vi "ReadDataUV-visSD_test.vi"(0 "Nombre de aq":i32=2, 1 "task out":refnum<k21> caption="tâche") -> (2 "Channel I":i32[][](array[numeric]), 3 "Channel II":i32[][](array[numeric]), 4 "DLL error code":u32=20066, 5 "temps d'acqu ms":u32=4148)   [LabVIEW 2015]
uses:
  dependecies/Error Code Enum typedef.ctl
  <vilib>/DAQmx/write.llb/DAQmx Write (Digital Bool 1Line 1Point).vi
panel:
  in  "Binning Horizontal":i32=1
  out "status":T1=enum."DRV_IDLE"
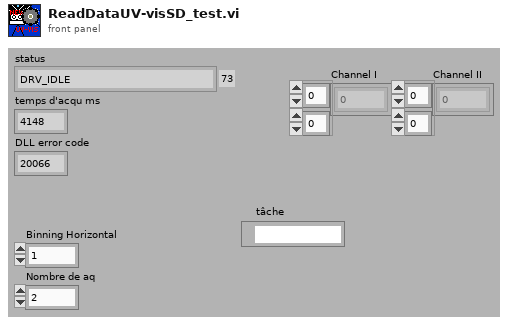
[diagram p1: front panel]
types:
  T1 = typedef "Error Code Enum typedef.ctl" = enum32{"N/A (0)", "DRV_ERROR_CODES", "DRV_SUCCESS", "DRV_VXDNOTINSTALLED", "DRV_ERROR_SCAN", "DRV_ERROR_CHECK_SUM", "DRV_ERROR_FILELOAD", "DRV_UNKNOWN_FUNC", "DRV_ERROR_VXD_INIT", "DRV_ERROR_ADDRESS", "DRV_ERROR_PAGELOCK", "DRV_ERROR_PAGEUNLOCK", "DRV_ERROR_BOARDTEST", "DRV_ERROR_ACK", "DRV_ERROR_UP_FIFO", "DRV_ERROR_PATTERN", "N/A (16)", "DRV_ACQUISITION_ERRORS", "DRV_ACQ_BUFFER", "DRV_ACQ_DOWNFIFO_FULL", "DRV_PROC_UNKONWN_INSTRUCTION", "DRV_ILLEGAL_OP_CODE", "DRV_KINETIC_TIME_NOT_MET", "DRV_ACCUM_TIME_NOT_MET", "DRV_NO_NEW_DATA", "N/A (25)", "DRV_SPOOLERROR", "N/A (27)", "N/A (28)", "N/A (29)", "N/A (30)", "N/A (31)", "N/A (32)", "DRV_TEMPERATURE_CODES", "DRV_TEMPERATURE_OFF", "DRV_TEMPERATURE_NOT_STABILIZED", "DRV_TEMPERATURE_STABILIZED", "DRV_TEMPERATURE_NOT_REACHED", "DRV_TEMPERATURE_OUT_RANGE", "DRV_TEMPERATURE_NOT_SUPPORTED", "DRV_TEMPERATURE_DRIFT", "N/A (41)", "N/A (42)", "N/A (43)", "N/A (44)", "N/A (45)", "N/A (46)", "N/A (47)", "N/A (48)", "DRV_GENERAL_ERRORS", "DRV_INVALID_AUX", "DRV_COF_NOTLOADED", "DRV_FPGAPROG", "DRV_FLEXERROR", "DRV_GPIBERROR", "N/A (55)", "N/A (56)", "N/A (57)", "N/A (58)", "N/A (59)", "N/A (60)", "N/A (61)", "N/A (62)", "N/A (63)", "DRV_DATATYPE", "DRV_DRIVER_ERRORS", "DRV_P1INVALID", "DRV_P2INVALID", "DRV_P3INVALID", "DRV_P4INVALID", "DRV_INIERROR", "DRV_COFERROR", "DRV_ACQUIRING", "DRV_IDLE", "DRV_TEMPCYCLE", "DRV_NOT_INITIALIZED", "DRV_P5INVALID", "DRV_P6INVALID", "DRV_INVALID_MODE", "DRV_INVALID_FILTER", "DRV_I2CERRORS", "DRV_I2CDEVNOTFOUND", "DRV_I2CTIMEOUT", "DRV_P7INVALID", "N/A (84)", "N/A (85)", "N/A (86)", "N/A (87)", "N/A (88)", "N/A (89)", "DRV_IOCERROR", "DRV_VRMVERSIONERROR"}
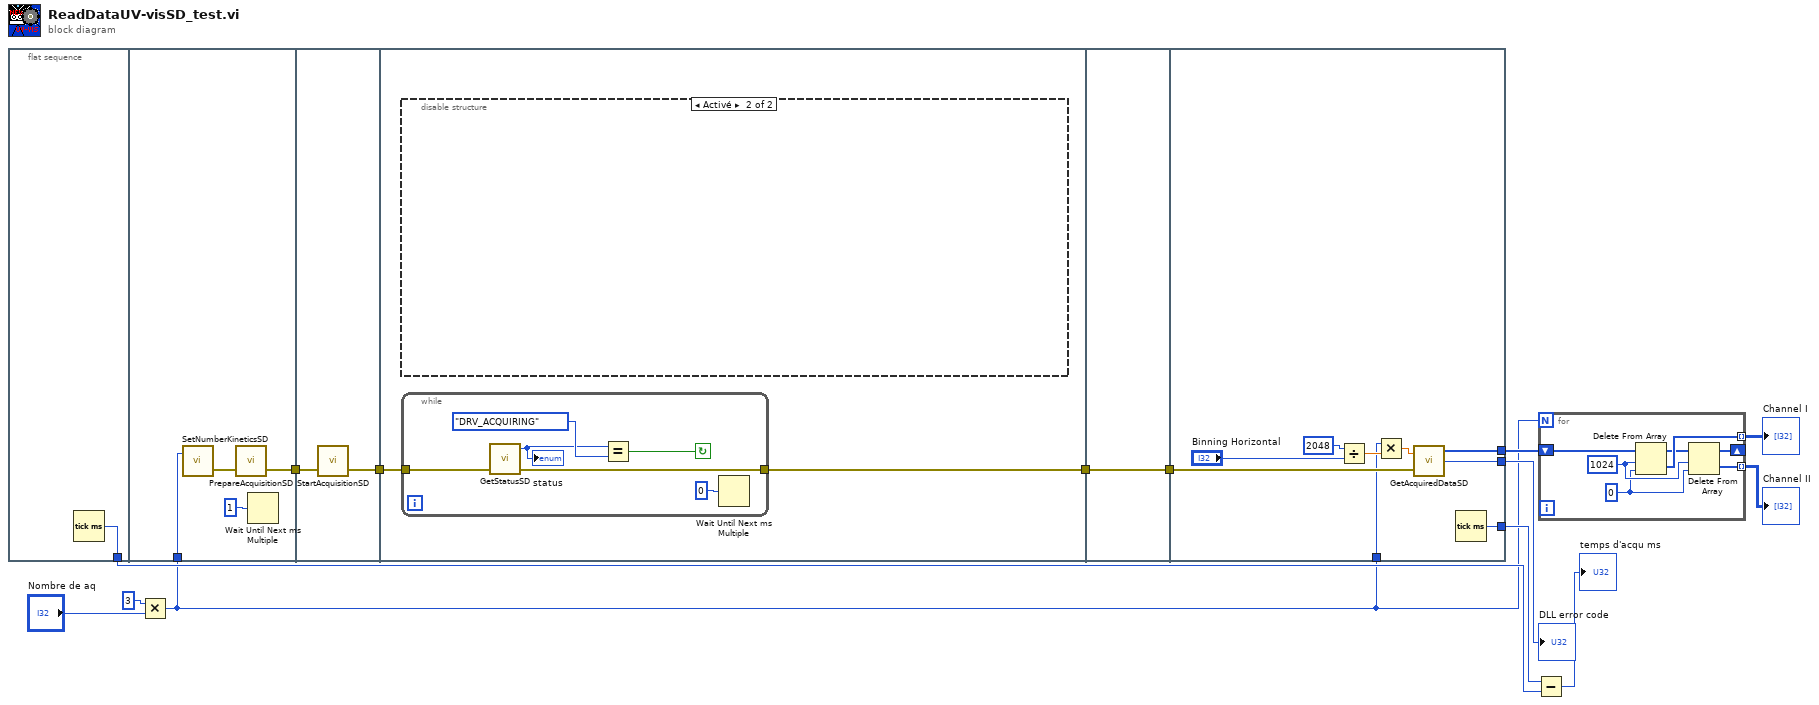
[diagram p0: block diagram]
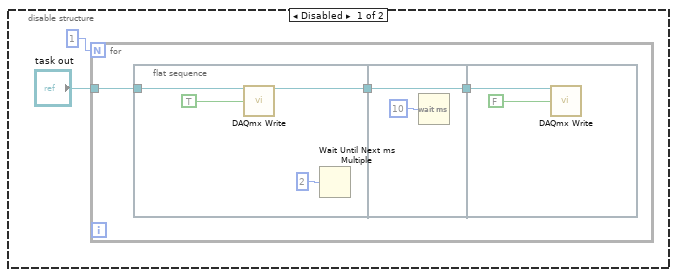
[diagram p2: hidden frame]
diagram:
  n1 = flat-sequence {
    tunnel: [w15] -> w10
    tunnel: [w17] -> w12
    tunnel: w2 -> [w16]
    tunnel: w12 -> [w21]
    tunnel: [w20] -> w11
    tunnel: w11 -> [w23]
    tunnel: [w22] -> w4
    tunnel: w4 -> [w43]
    tunnel: [w43] -> w3
    tunnel: [w51] -> w8
    tunnel: [w50] -> w14
    tunnel: w3 -> [w47]
    tunnel: [w46] -> w9
    tunnel: w2 -> [w45]
    frame #0 {
      n2 = Tick Count (ms)() -> (millisecond timer value=w15:u32)
    }
    frame #1 {
      n3 = call "SetNumberKineticsSD.vi"("number"=w16) -> ("error out"=w19:errorcluster)  [unwired: 1 in, 1 out]
      n4 = call "PrepareAcquisitionSD.vi"("error in (no error)"=w19) -> ("error out"=w17:errorcluster)  [unwired: 1 in, 1 out]
      n5 = Wait Until Next ms Multiple(millisecond multiple=u32 1 ("n millisecondes")) -> ()  [unwired: 1 out]
    }
    frame #2 {
      n6 = call "StartAcquisitionSD.vi"("error in (no error)"=w21) -> ("error out"=w20:errorcluster)  [unwired: 1 in, 1 out]
    }
    frame #3 {
      n7 = disable-structure shown="Activé" {
        frame Disabled {
          n8 = for {
            N: 1 -> [_]
            tunnel: "task out" -> [w28]
            n9 = flat-sequence {
              tunnel: w28 -> [w32]
              tunnel: [w30] -> w26
              tunnel: [w33] -> w27
              tunnel: w26 -> [w33]
              tunnel: w27 -> [w36]
              frame #0 {
                n10 = call-poly <vilib>:"DAQmx Write.vi"("task/channels in"=w32, "data"=TRUE) -> ("task out"=w30:refnum<k21>)  [unwired: 11 in, 2 out]
                n11 = Wait Until Next ms Multiple(millisecond multiple=u32 2 ("n millisecondes")) -> ()  [unwired: 1 out]
              }
              frame #1 {
                n12 = Wait (ms)(milliseconds to wait=u32 10 ("n millisecondes")) -> ()  [unwired: 1 out]
              }
              frame #2 {
                n13 = call-poly <vilib>:"DAQmx Write.vi"("task/channels in"=w36, "data"=FALSE) -> ()  [unwired: 11 in, 3 out]
              }
            }
          }
        }
        frame Enabled {
        }
      }
      n14 = while {
        tunnel: w23 -> [w39]
        tunnel: [w38] -> w22
        stop <- w41 continue-if-true
        n15 = call "GetStatusSD.vi"("error in (no error)"=w39) -> ("error out"=w38:errorcluster, "status"=w40:T1)  [unwired: 2 in, 1 out]
        "status" <- w40
        n16 = Equal?(x=w40, y=Error_Code_Enum_typedef."DRV_ACQUIRING") -> (x = y?=w41:bool)
        n17 = Wait Until Next ms Multiple(millisecond multiple=u32 0 ("n millisecondes")) -> ()  [unwired: 1 out]
      }
    }
    frame #4 {
    }
    frame #5 {
      n18 = Divide(x=2048 ("y"), y="Binning Horizontal") -> (x/y=w49:dbl)
      n19 = Multiply(x=w45, y=w49) -> (x*y=w52:dbl)
      n20 = call "GetAcquiredDataSD.vi"("size"=w52, "error in (no error)"=w47) -> ("array"=w51:i32[], "DLL error code"=w50:u32)  [unwired: 1 out]
      n21 = Tick Count (ms)() -> (millisecond timer value=w46:u32)
    }
  }
  n22 = Multiply(x=3, y="Nombre de aq") -> (x*y=w2:i32)
  n23 = Subtract(x=w9, y=w10) -> (x-y=→"temps d'acqu ms":u32)
  n24 = for {
    N: w2 -> [_]
    shift-right: [w53] -> _
    shift-left: w8 -> [w59]
    tunnel: [w58] -> w7 mode=indexing
    tunnel: [w54] -> w6 mode=indexing
    w55 = 0 ("index")
    w56 = 1024 ("length")
    n25 = Delete From Array(array=w59, length=w56, index=w55) -> (deleted portion=w58:i32[], array with subset deleted=w57:i32[])
    n26 = Delete From Array(array=w57, length=w56, index=w55) -> (deleted portion=w54:i32[], array with subset deleted=w53:i32[])
  }
  "Channel I" <- w7
  "Channel II" <- w6
  "DLL error code" <- w14
